vi "Create Interaction information channels (outgoing).vi"(8 "error in":errorcluster, 11 "Item Ref in":T1 format="%.0x") -> (0 "error out":errorcluster, 3 "Item Ref out":T1 format="%.0x")   [LabVIEW 2019, in "HLA Custom Device System Explorer.lvlib"]
uses:
  HLA Custom Device System Explorer.lvlib
  <vilib>/NI VeriStand/Custom Device API/Custom Device Item Ref.ctl
  <vilib>/NI VeriStand/Custom Device API/Custom Device Channel.ctl
  <vilib>/NI VeriStand/Custom Device API/Custom Device Channel Type.ctl
  <vilib>/NI VeriStand/Custom Device API/Custom Device API.lvlib
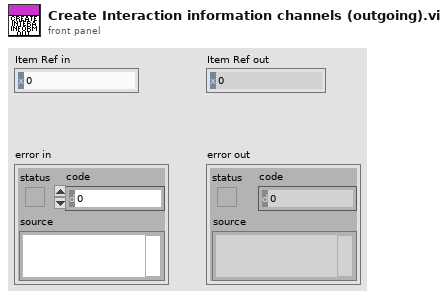
[diagram p1: front panel]
types:
  T1 = typedef "Custom Device API.lvlib/Custom Device Item Ref.ctl" = u64
  T2 = typedef "Custom Device API.lvlib/Custom Device Channel.ctl" = cluster{"Type":T3, "Units":string, "Default Value":dbl, "Faultable":bool, "Scalable":bool}
  T3 = typedef "Custom Device API.lvlib/Custom Device Channel Type.ctl" = enum16{"Input", "Output"}
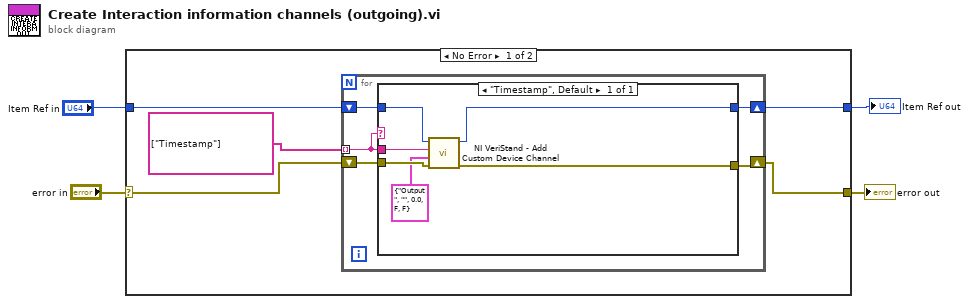
[diagram p0: block diagram]
diagram:
  n1 = case shown="No Error" "error in" {
    selector: "error in" -> [w7 w21]
    tunnel: [w6 w21] -> w3
    tunnel: [w8 w22] -> w2
    tunnel: "Item Ref in" -> [w9 w22]
    frame No Error {
      n2 = for {
        shift-right: [w13] -> w8
        shift-left: w9 -> [w14]
        shift-right: [w11] -> w6
        shift-left: w7 -> [w12]
        tunnel: string[] ["Timestamp"] -> [w10] mode=indexing
        n3 = case shown="\"Timestamp\", Default" w10 {
          tunnel: w14 -> [w20]
          tunnel: [w19] -> w13
          tunnel: w12 -> [w18]
          tunnel: [w17] -> w11
          tunnel: w10 -> [w16]
          frame "Timestamp", Default {
            n4 = call <vilib>:"NI VeriStand - Add Custom Device Channel.vi"("error in (no error)"=w18, "Channel"=T2 {"Type"=enum."Output", "Units"="", "Default Value"=0.0, "Faultable"=FALSE, "Scalable"=FALSE}, "Channel Name"=w16, "Parent Ref in"=w20) -> ("error out"=w17:errorcluster, "Parent Ref out"=w19:T1)  [unwired: 4 in, 2 out]
          }
        }
      }
    }
    frame Error {
    }
  }
  "error out" <- w3
  "Item Ref out" <- w2
